vi "Sequencer.mqtt.vi"() -> ()   [LabVIEW 2014]
uses:
  <vilib>/daq.io/MQTT LabVIEW Client/Controls/Connection_Return_Codes.ctl
  <vilib>/addons/zeromq/socket_type.ctl
  <vilib>/daq.io/MQTT LabVIEW Client/Controls/Connect_Flags.ctl
  <vilib>/daq.io/MQTT LabVIEW Client/Controls/QoS.ctl
  <vilib>/daq.io/MQTT LabVIEW Client/Controls/DUP_Flag.ctl
  <vilib>/daq.io/MQTT LabVIEW Client/Controls/Retain_Flag.ctl
  <vilib>/Analysis/NI_AALPro.lvlib
  <vilib>/addons/zeromq/zmq_context.lvclass
  <vilib>/addons/zeromq/zmq_socket.lvclass
  <vilib>/addons/zeromq/zeromq.lvlib
  <vilib>/daq.io/MQTT LabVIEW Client/MQTT_Functions.lvlib
panel:
  out "MQTT Error":string
  out "MQTT Status":T1=enum."Connection refused: not authorized"
  out "Counts":u32[](array[numeric])
  out "PMT4":u32[](array[numeric])
  out "PMT3":u32[](array[numeric])
  out "PMT2":u32[](array[numeric])
  out "PMT1":u32[](array[numeric])
  in  "Threshold":dbl=1.0
  out "CompiledSequence":string="#DopplerCooling\r\n0.9 10100000 00000000 00000000\r\n\r\n#Pump\r\n0.3 01000000 00000000 00000000\r\n\r\n#Pulsed\r\n0.2 00100000 00000000 00000000\r\n0.4 00000100 00000000 00000000\r\n0.2 00000000 10000000 00000000\r\n0.2 01000000 00000000 01000000\n"
  out "ChapterNames":string[](array[string])
  out "ChapterPositions":u32[](array[numeric])
  in  "Scan":enum32{"Time"}(tab)
  out "Now (us)":dbl=1.0 format="%.2f"
  in  "Step (us)":dbl=1.0 format="%.2f"
  in  "End (us)":dbl=1.0 format="%.2f"
  in  "Start (us)":dbl=1.0 format="%.2f"
  in  "Time Scan":bool
  in  "Chapter":u16(ring) items=["Zero", "DopplerCooling[0]", "DopplerCooling[1]", "DopplerCooling[2]", "Zero"]
  in  "Once":bool=TRUE
  in  "Sequencer Port":refnum<visa-resource-name>="COM8"
  in  "Send":bool
  out "Durations Backup":dbl[](array[numeric])
  out "Durations":dbl[](array[numeric])
  in  "Period (ns)":dbl=5.0
  out "States":string[](array[string])
  in  "Sequencer":bool
  in  "Edit":enum32{"Sequence"}(tab)
  in  "Sequence":string
  in  "Save":bool
  in  "Chapter (us)":string
  in  "Sequence File":path=path "D:/Data/Sequence/Cooling.seq"
  in  "Repeats":u32=100
  in  "Compile":bool
  in  "Data":bool
  out "Clock":string
  in  "Detect":enum32{"PMT", "TTL"}(tab)
  in  "4":bool
  in  "3":bool
  in  "2":bool
  in  "1":bool=TRUE
  in  "Save":bool
  in  "Count or State":i16(ring) items=["Count", "State"]
  in  "Fit":bool
  out "Peak":u32
  out "?":cluster{dbl[], "Axis":dbl[]}(graph)
  out "?":cluster{"Axis":dbl[], "Histogram":i32[]}(graph)
  in  "Data Chapter":i16(ring) items=["All", "DopplerCooling[2]"]
  out "Average Counts or States":dbl(graph)
  out "Average of Scans":dbl[](graph)
  out "data file":string
  out "History Data":dbl[](array[numeric])
  in  "Sweep":bool
  out "Digital Waveform Graph":digitaldata(graph)
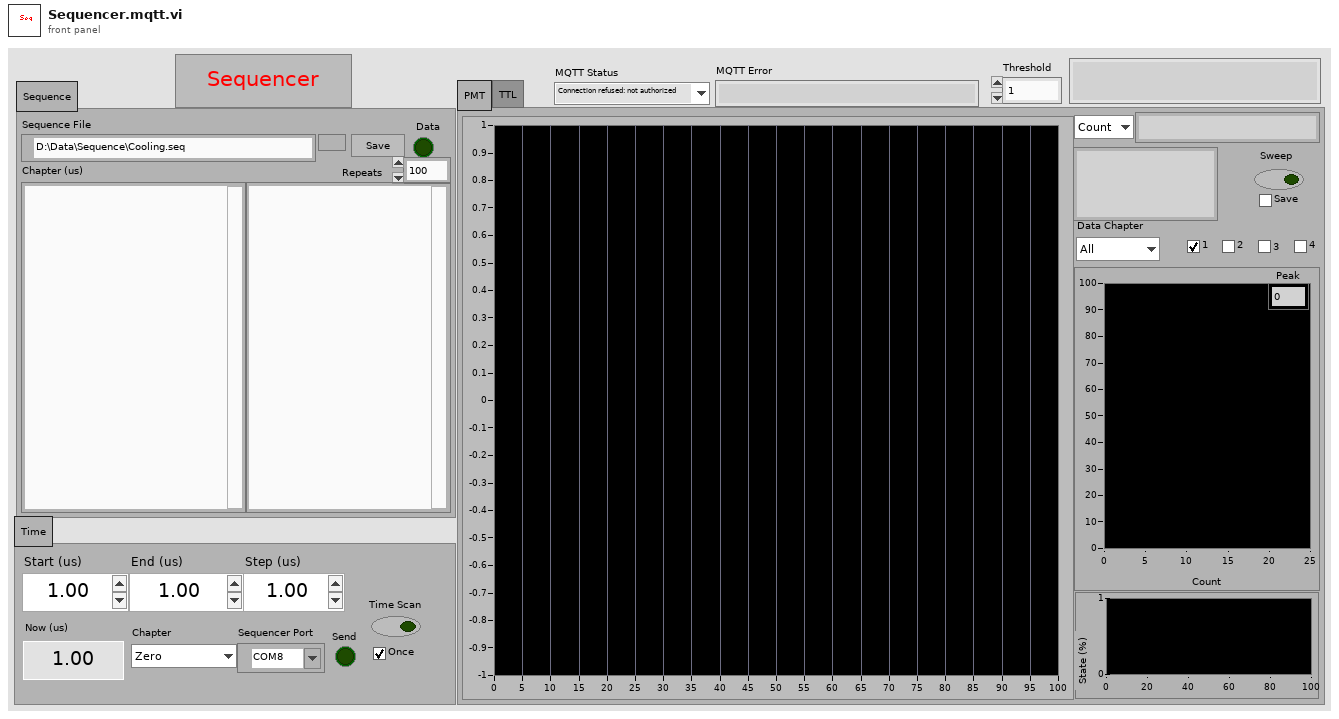
[diagram p1: front panel]
types:
  T1 = typedef "MQTT_Functions.lvlib/Connection_Return_Codes.ctl" = enum16{"Connection accepted", "Connection refused: unacceptable protocol version", "Connection refused: identifier rejected", "Connection refused: Server unavailable", "Connection refused: bad user name or password", "Connection refused: not authorized"}
  T2 = typedef "MQTT_Functions.lvlib/QoS.ctl" = enum8{"At most once", "At least once", "Exactly once", "Reserved"}
  T3 = typedef "MQTT_Functions.lvlib/DUP_Flag.ctl" = bool
  T4 = typedef "MQTT_Functions.lvlib/Retain_Flag.ctl" = bool
  T5 = cluster{"QoS":T2, "DUP":T3, "Retain":T4, "Keep Alive (sec)":u16}
  T6 = typedef "MQTT_Functions.lvlib/Connect_Flags.ctl" = cluster{"user name":bool, "password":bool, "will retain":bool, "will flag":bool, "clean session":bool, "reserved":bool, "will QoS":T2}
  T7 = typedef "zeromq.lvlib/socket_type.ctl" = enum8{"ZMQ_PAIR", "ZMQ_PUB", "ZMQ_SUB", "ZMQ_REQ", "ZMQ_REP", "ZMQ_DEALER", "ZMQ_ROUTER", "ZMQ_PULL", "ZMQ_PUSH", "ZMQ_XPUB", "ZMQ_XSUB"}
  T8 = cluster{"lower":dbl, "upper":dbl, "inclusion":enum32{"lower", "upper", "both", "neither"}}[]
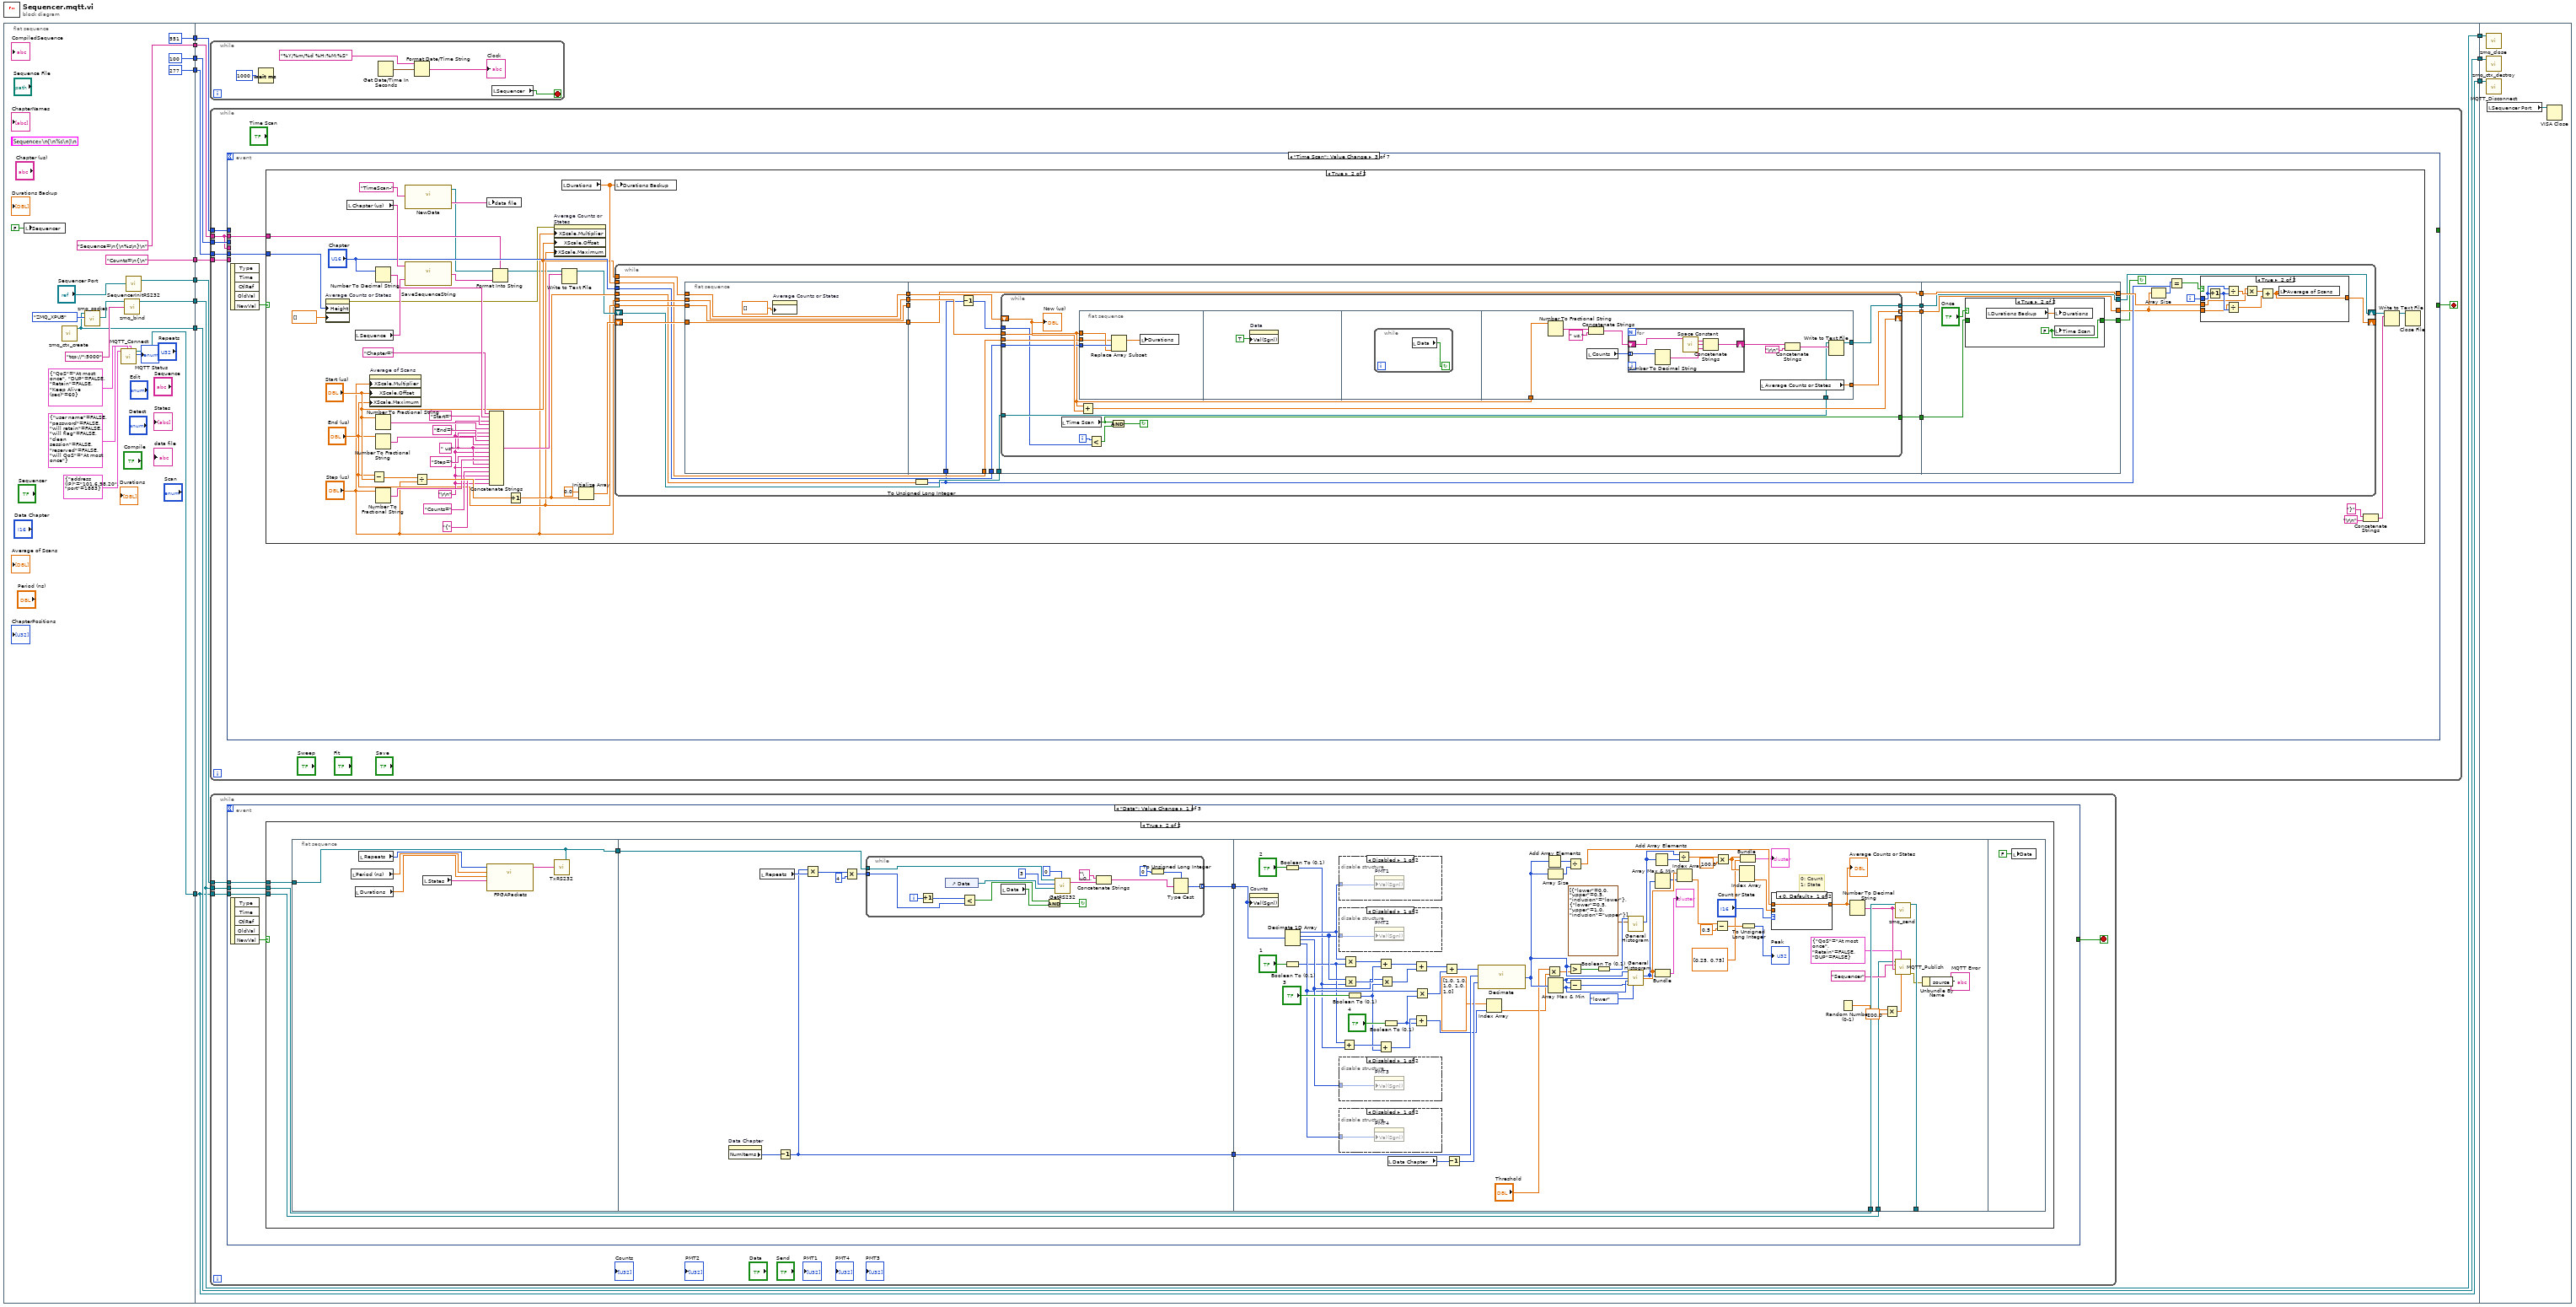
[diagram p0: block diagram]
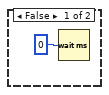
[diagram p2: hidden frame]
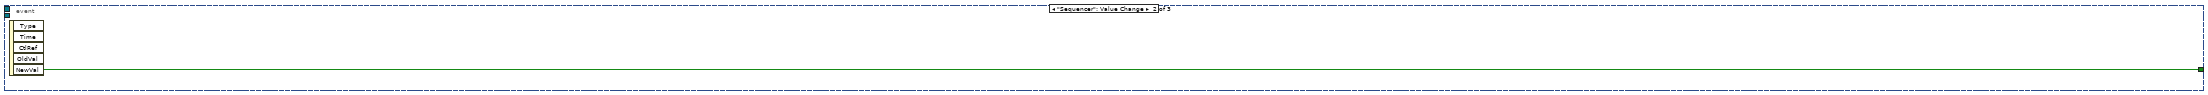
[diagram p8: hidden frame]
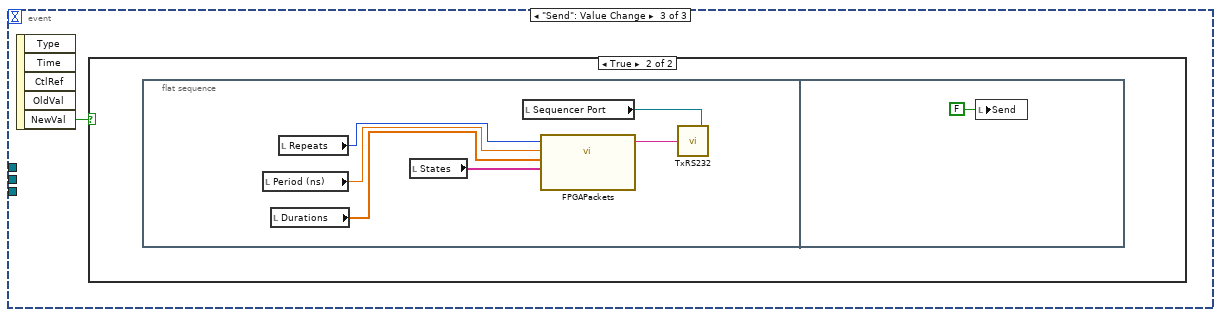
[diagram p9: hidden frame]
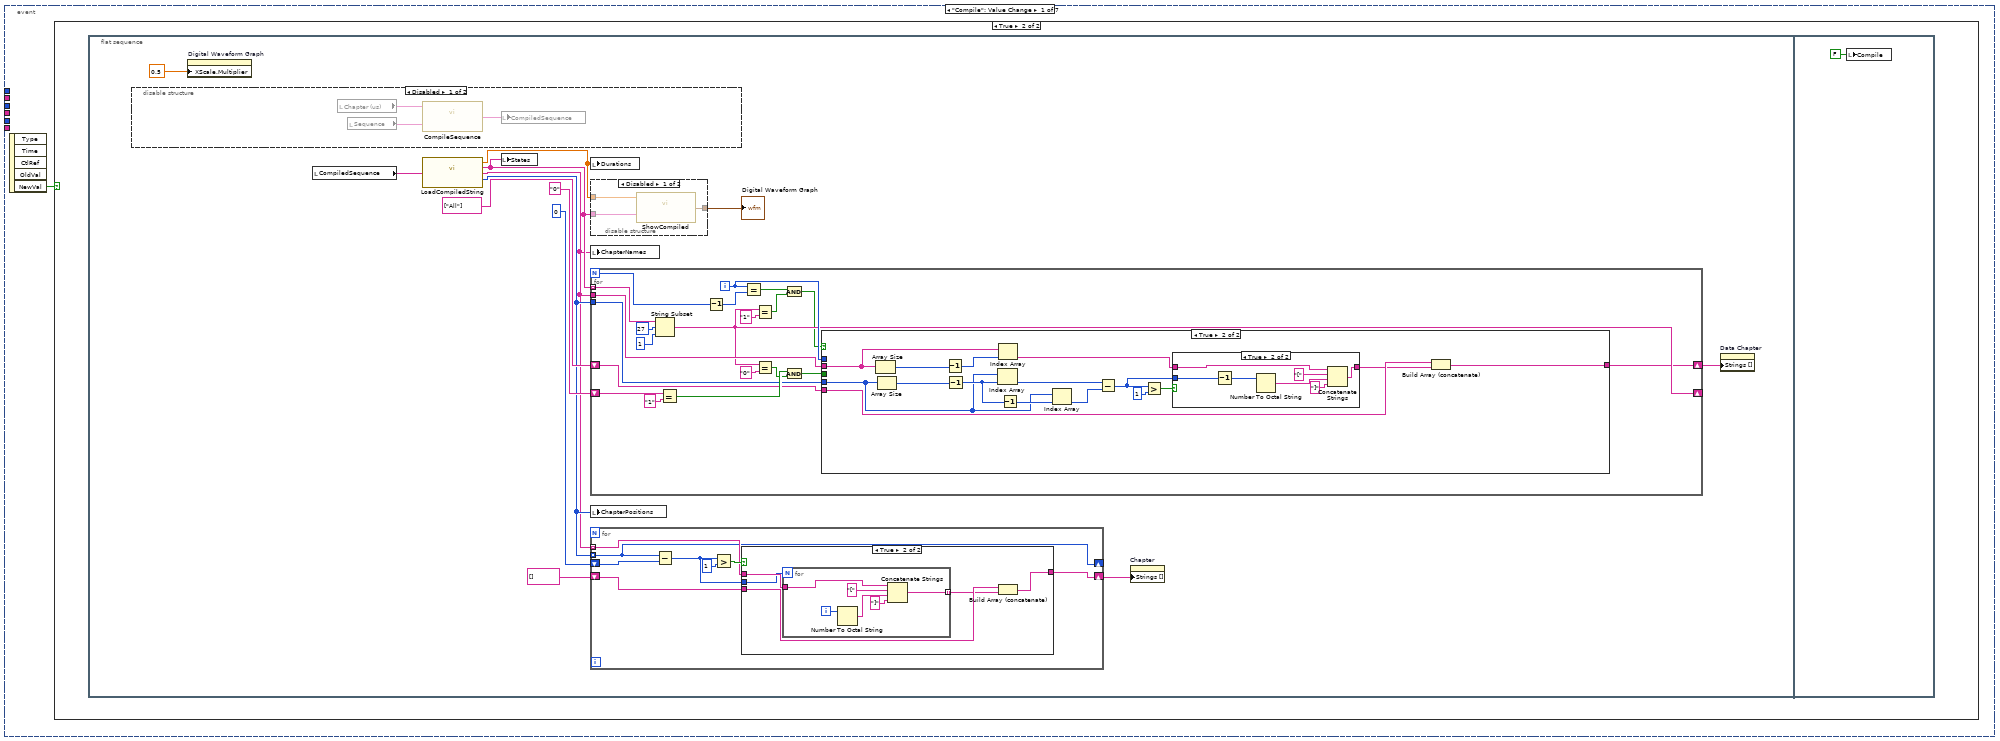
[diagram p11: hidden frame]
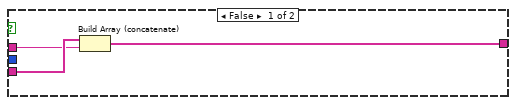
[diagram p15: hidden frame]
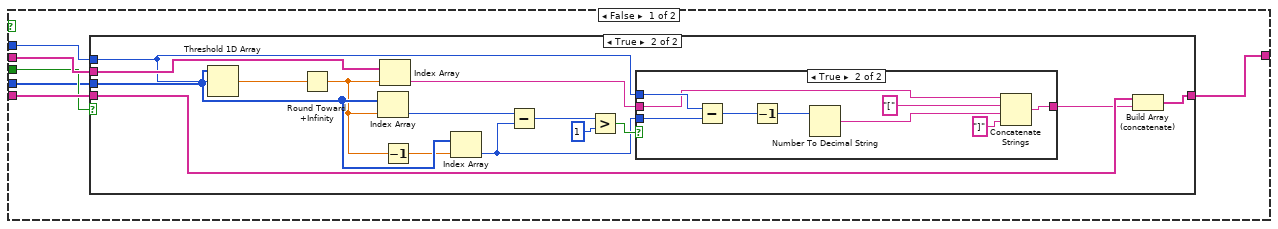
[diagram p16: hidden frame]
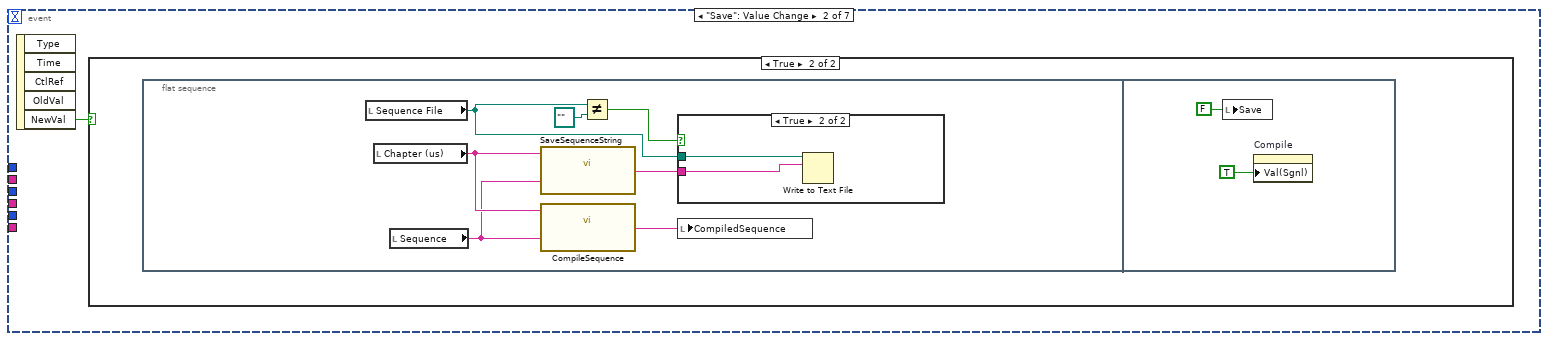
[diagram p20: hidden frame]
diagram:
  n1 = flat-sequence {
    tunnel: [w23] -> w12
    tunnel: [u32 277 ("XControl:Container Bounds:Height")] -> w11
    tunnel: [u32 551 ("Plot Area:Size:Height")] -> w10
    tunnel: [100 ("y")] -> w9
    tunnel: ["Sequence=\n{\n%s\n}\n" ("format string")] -> w8
    tunnel: ["Counts=\n{\n" ("text")] -> w7
    tunnel: [w19] -> w6
    tunnel: [w18] -> w3
    tunnel: [w16] -> w2
    tunnel: w12 -> [w39]
    tunnel: w11 -> [w38]
    tunnel: w10 -> [w37]
    tunnel: w9 -> [w36]
    tunnel: w8 -> [w35]
    tunnel: w7 -> [w34]
    tunnel: w6 -> [w32]
    tunnel: [w32] -> w5
    tunnel: [w33] -> w4
    tunnel: w3 -> [w33]
    tunnel: w2 -> [w31]
    tunnel: [w31] -> w1
    tunnel: w5 -> [w534]
    tunnel: w4 -> [w533]
    tunnel: w1 -> [w532]
    frame #0 {
      n2 = local write "Sequencer"(FALSE ("Sequencer")) -> ()
      n3 = call <vilib>:"zmq_ctx_create.vi"() -> ("context out"=w18:refnum<class "zmq_context.lvclass">)  [unwired: 4 in, 1 out]
      n4 = call <vilib>:"zmq_socket.vi"("socket type"=socket_type."ZMQ_XPUB", "context in"=w18) -> ("socket out"=w21:refnum<class "zmq_socket.lvclass">)  [unwired: 3 in, 2 out]
      n5 = call <vilib>:"MQTT_Connect.vi"("Connect Meta"=T5 {"QoS"=enum."At most once", "DUP"=FALSE, "Retain"=FALSE, "Keep Alive (sec)"=60}, "Connect Flags"=T6 {"user name"=FALSE, "password"=FALSE, "will retain"=FALSE, "will flag"=FALSE, "clean session"=FALSE, "reserved"=FALSE, "will QoS"=enum."At most once"}, "MQTT Broker"=cluster{"address (IP)":string, "port":u16} {"address (IP)"="101.6.98.20", "port"=1883}) -> ("Connection Status"=→"MQTT Status":T1, "connection ID out"=w16:refnum<k5>)  [unwired: 6 in, 1 out]
      n6 = call <vilib>:"zmq_bind.vi"("endpoint"="tcp://*:5000", "socket in"=w21) -> ("socket out"=w19:refnum<class "zmq_socket.lvclass">)  [unwired: 2 in, 1 out]
      n7 = call "SequencerInitRS232.vi"("VISA resource name"="Sequencer Port") -> ("reference out"=w23:refnum<visa-resource-name>)  [unwired: 1 out]
    }
    frame #1 {
      n8 = while {
        stop <- w40 stop-if-true
        n9 = Wait (ms)(milliseconds to wait=u32 1000) -> ()  [unwired: 1 out]
        n10 = Get Date/Time In Seconds() -> (seconds since 1Jan1904=w44:timestamp)
        n11 = Format Date/Time String(time format string (%c)="%Y/%m/%d %H:%M:%S", seconds (now)=w44) -> (date/time string=→"Clock":string)  [unwired: 1 in]
        n12 = local read "Sequencer"() -> (w40:bool)
      }
      n13 = while {
        tunnel: w38 -> [w180]
        tunnel: w37 -> [w179]
        tunnel: w36 -> [w178]
        tunnel: w35 -> [w176]
        tunnel: w34 -> [w177]
        stop <- w181 stop-if-true
        n14 = event shown="[2] \"Time Scan\": Value Change" {
          selector: _ -> [_ _ _ _ _ _ _]
          dyn-events: _ -> [_ _ _ _ _ _ _]
          timeout: _ -> [_ _ _ _ _ _ _]
          tunnel: [_ _ _ _ _ _ w531] -> _
          tunnel: [_ _ _ _ _ _ w531] -> w181
          tunnel: w180 -> [_ _ w315 _ _ _ _]
          tunnel: w179 -> [_ _ _ _ _ w468 _]
          tunnel: w178 -> [_ _ _ _ _ w467 _]
          tunnel: w176 -> [_ _ _ _ _ w466 _]
          tunnel: w177 -> [_ _ _ _ _ w465 _]
          tunnel: w176 -> [_ _ w314 _ _ _ _]
          event "Compile": Value Change {
            n15 = event-data() -> ("NewVal"=w182:bool)  [unwired: 1 in, 4 out]
            n16 = case shown="True" w182 {
              frame False {
              }
              frame True {
                n17 = flat-sequence {
                  frame #0 {
                    n18 = disable-structure shown="Disabled" {
                      frame Disabled {
                        n19 = local read "Chapter (us)"() -> (w201:string)
                        n20 = local read "Sequence"() -> (w200:string)
                        n21 = call "CompileSequence.vi"("Sequence"=w200, "Chapter"=w201) -> ("Compiled Sequence"=w199:string)
                        n22 = local write "CompiledSequence"(w199) -> ()
                      }
                      frame Enabled {
                      }
                    }
                    n23 = property on="Digital Waveform Graph" class="DigitalGraph (strict)"("XScale.Multiplier"=0.5 ("X Scale.Offset and Multiplier:Multiplier")) -> ()  [unwired: 2 in, 2 out]
                    n24 = local read "CompiledSequence"() -> (w183:string)
                    n25 = call "LoadCompiledString.vi"("Compiled String"=w183) -> ("Durations"=w194:dbl[], "States"=w193:string[], "ChapterNames"=w184:string[], "ChapterPositions"=w185:u32[])
                    n26 = local write "States"(w193) -> ()
                    n27 = local write "Durations"(w194) -> ()
                    n28 = disable-structure shown="Disabled" {
                      disable-tunnel: [w198 _] -> w195
                      disable-tunnel: w194 -> [w197 _]
                      disable-tunnel: w193 -> [w196 _]
                      frame Disabled {
                        n29 = call "ShowCompiled.vi"("States"=w196, "Durations"=w197) -> ("Digital Waveform Graph"=w198:digitaldata)
                      }
                      frame Enabled {
                      }
                    }
                    "Digital Waveform Graph" <- w195
                    n30 = local write "ChapterNames"(w184) -> ()
                    n31 = for {
                      N -> [w235]
                      tunnel: w193 -> [w244] mode=indexing
                      shift-right: [w232] -> _
                      shift-left: "0" -> [w242]
                      tunnel: w184 -> [w238]
                      shift-right: [w227] -> w188
                      shift-left: string[] ["All"] -> [w226]
                      tunnel: w185 -> [w225]
                      i -> [w236]
                      n32 = String Subset(string=w244, offset (0)=27, length (rest)=1 ("length (rest)")) -> (substring=w232:string)
                      n33 = Equal?(x=w242, y="1") -> (x = y?=w240:bool)
                      n34 = Decrement(x=w235) -> (x-1=w234:i32)
                      n35 = Equal?(x=w236, y=w234) -> (x = y?=w231:bool)
                      n36 = Equal?(x=w232, y="1") -> (x = y?=w230:bool)
                      n37 = Equal?(x=w232, y="0") -> (x = y?=w237:bool)
                      n38 = And(x=w231, y=w230) -> (x .and. y?=w229:bool)
                      n39 = And(x=w240, y=w237) -> (x .and. y?=w228:bool)
                      n40 = case shown="True" w229 {
                        tunnel: w238 -> [w250 w290]
                        tunnel: w226 -> [w249 w292]
                        tunnel: w236 -> [w248 _]
                        tunnel: w228 -> [w247 _]
                        tunnel: [w246 w291] -> w227
                        tunnel: w225 -> [w245 w284]
                        frame False {
                          n41 = case shown="True" w247 {
                            tunnel: w248 -> [_ w262]
                            tunnel: w250 -> [_ w263]
                            tunnel: w249 -> [w251 w265]
                            tunnel: [w251 w266] -> w246
                            tunnel: w245 -> [_ w259]
                            frame False {
                            }
                            frame True {
                              n42 = Threshold 1D Array(2:w262, 3:w259) -> (0:w264:dbl)  [unwired: 1 in]
                              n43 = Round Toward +Infinity(x=w264) -> (ceil(x): smallest int >= x=w257:dbl)
                              n44 = Index Array(array=w259, index=w257) -> (element=w256:u32)
                              n45 = Index Array(array=w263, index=w257) -> (element=w260:string)
                              n46 = Decrement(x=w257) -> (x-1=w258:dbl)
                              n47 = Index Array(array=w259, index=w258) -> (element=w252:u32)
                              n48 = Subtract(x=w256, y=w252) -> (x-y=w255:u32)
                              n49 = Greater?(x=w255, y=u32 1) -> (0:w253:bool)
                              n50 = case shown="True" w253 {
                                tunnel: w262 -> [_ w276]
                                tunnel: [w267 w270] -> w261
                                tunnel: w260 -> [w267 w269]
                                tunnel: w252 -> [_ w268]
                                frame False {
                                }
                                frame True {
                                n51 = Subtract(x=w276, y=w268) -> (x-y=w275:u32)
                                n52 = Decrement(x=w275) -> (x-1=w274:u32)
                                n53 = Number To Decimal String(number=w274) -> (decimal integer string=w271:string)  [unwired: 1 in]
                                n54 = Concatenate Strings(w269, "[" ("element"), w271, "]" ("element")) -> (w270:string)
                                }
                              }
                              n55 = Build Array (concatenate)(w265, w261) -> (w266:string[])
                            }
                          }
                        }
                        frame True {
                          n56 = Array Size(array=w290) -> (size(s)=w289:i32)
                          n57 = Array Size(array=w284) -> (size(s)=w287:i32)
                          n58 = Decrement(x=w289) -> (x-1=w288:i32)
                          n59 = Decrement(x=w287) -> (x-1=w286:i32)
                          n60 = Index Array(array=w284, index=w286) -> (element=w283:u32)
                          n61 = Index Array(array=w290, index=w288) -> (element=w279:string)
                          n62 = Decrement(x=w286) -> (x-1=w285:i32)
                          n63 = Index Array(array=w284, index=w285) -> (element=w282:u32)
                          n64 = Subtract(x=w283, y=w282) -> (x-y=w277:u32)
                          n65 = Greater?(x=w277, y=u32 1) -> (0:w280:bool)
                          n66 = case shown="True" w280 {
                            tunnel: w279 -> [w293 w300]
                            tunnel: [w293 w294] -> w278
                            tunnel: w277 -> [_ w297]
                            frame False {
                            }
                            frame True {
                              n67 = Decrement(x=w297) -> (x-1=w296:u32)
                              n68 = Number To Octal String(2:w296) -> (0:w295:string)  [unwired: 1 in]
                              n69 = Concatenate Strings(w300, "[" ("string"), w295, "]" ("string")) -> (w294:string)
                            }
                          }
                          n70 = Build Array (concatenate)(w292, w278) -> (w291:string[])
                        }
                      }
                    }
                    n71 = local write "ChapterPositions"(w185) -> ()
                    n72 = for {
                      tunnel: w185 -> [w202] mode=indexing
                      tunnel: w184 -> [w203] mode=indexing
                      shift-right: [w202] -> _
                      shift-left: u32 0 ("initial scan location") -> [w209]
                      shift-right: [w204] -> w190
                      shift-left: string[] [] -> [w205]
                      n73 = Subtract(x=w202, y=w209) -> (x-y=w206:u32)
                      n74 = Greater?(x=w206, y=u32 1) -> (0:w208:bool)
                      n75 = case shown="True" w208 {
                        tunnel: w203 -> [w211 w217]
                        tunnel: w206 -> [_ w216]
                        tunnel: w205 -> [w212 w215]
                        tunnel: [w210 w213] -> w204
                        frame False {
                          n76 = Build Array (concatenate)(w212, w211) -> (w210:string[])
                        }
                        frame True {
                          n77 = for {
                            N: w216 -> [_]
                            tunnel: w217 -> [w222]
                            tunnel: [w221] -> w214 mode=indexing
                            i -> [w223]
                            n78 = Number To Octal String(2:w223) -> (0:w220:string)  [unwired: 1 in]
                            n79 = Concatenate Strings(w222, "[" ("string"), w220, "]" ("string")) -> (w221:string)
                          }
                          n80 = Build Array (concatenate)(w215, w214) -> (w213:string[])
                        }
                      }
                    }
                    n81 = property on="Chapter" class="Ring (strict)"("Strings []"=w190) -> ()  [unwired: 2 in, 2 out]
                    n82 = property on="Data Chapter" class="Ring (strict)"("Strings []"=w188) -> ()  [unwired: 2 in, 2 out]
                  }
                  frame #1 {
                    n83 = local write "Compile"(FALSE ("Compile")) -> ()
                  }
                }
              }
            }
          }
          event "Save": Value Change {
            n84 = event-data() -> ("NewVal"=w302:bool)  [unwired: 1 in, 4 out]
            n85 = case shown="True" w302 {
              frame False {
              }
              frame True {
                n86 = flat-sequence {
                  frame #0 {
                    n87 = local read "Sequence File"() -> (w307:path)
                    n88 = local read "Chapter (us)"() -> (w305:string)
                    n89 = local read "Sequence"() -> (w304:string)
                    n90 = call "SaveSequenceString.vi"("Sequence"=w304, "Chapter"=w305) -> ("Sequence String"=w306:string)
                    n91 = call "CompileSequence.vi"("Sequence"=w304, "Chapter"=w305) -> ("Compiled Sequence"=w303:string)
                    n92 = Not Equal?(x=w307, y=path "") -> (x != y?=w309:bool)
                    n93 = case shown="True" w309 {
                      tunnel: w307 -> [_ w311]
                      tunnel: w306 -> [_ w310]
                      frame False {
                      }
                      frame True {
                        n94 = Write to Text File(file (use dialog)=w311, text=w310) -> ()  [unwired: 2 in, 3 out]
                      }
                    }
                    n95 = local write "CompiledSequence"(w303) -> ()
                  }
                  frame #1 {
                    n96 = local write "Save"(FALSE ("Compile")) -> ()
                    n97 = property on="Compile" class="Bool (strict)"("Val(Sgnl)"=TRUE ("Value (Signaling)")) -> ()  [unwired: 2 in, 2 out]
                  }
                }
              }
            }
          }
          event "Time Scan": Value Change {
            n98 = event-data() -> ("NewVal"=w316:bool)  [unwired: 1 in, 4 out]
            n99 = case shown="True" w316 {
              tunnel: w315 -> [_ w328]
              tunnel: w314 -> [_ w321]
              frame False {
                n100 = local read "Durations Backup"() -> (w317:dbl[])
                n101 = local write "Durations"(w317) -> ()
              }
              frame True {
                w341 = " us" ("string")
                w338 = "\r\n"
                n102 = property on="Average Counts or States" class="WFChart (strict)"("Height"=w328, "History Data"=dbl[] []) -> (error out=w327:errorcluster)  [unwired: 2 in, 1 out]
                n103 = local read "Chapter (us)"() -> (w348:string)
                n104 = local read "Sequence"() -> (w349:string)
                n105 = property on="Average of Scans" class="WFGraph (strict)"("XScale.Multiplier"="Step (us)", "XScale.Offset"="Start (us)", "XScale.Maximum"="End (us)") -> ()  [unwired: 2 in, 2 out]
                n106 = Subtract(x="End (us)", y="Start (us)") -> (x-y=w356:dbl)
                n107 = Number To Decimal String(number="Chapter") -> (decimal integer string=w352:string)  [unwired: 1 in]
                n108 = Number To Fractional String(number="Start (us)") -> (F-format string=w346:string)  [unwired: 3 in]
                n109 = Number To Fractional String(number="End (us)") -> (F-format string=w344:string)  [unwired: 3 in]
                n110 = Number To Fractional String(number="Step (us)") -> (F-format string=w342:string)  [unwired: 3 in]
                n111 = call "NewData.vi"("Prefix"="TimeScan-" ("string")) -> ("data file name"=w325:string, "data file refnum"=w319:refnum<file>)  [unwired: 2 in]
                n112 = call "SaveSequenceString.vi"("Sequence"=w349, "Chapter"=w348) -> ("Sequence String"=w320:string)
                n113 = Divide(x=w356, y="Step (us)") -> (x/y=w355:dbl)
                n114 = local write "data file"(w325) -> ()
                n115 = Concatenate Strings("Chapter=" ("string"), w352, w338, "Start=" ("string"), w346, w341, w338, "End=" ("string"), w344, w341, w338, "Step=" ("string"), w342, w341, w338, "Counts=" ("string"), w338, "{" ("string"), w338) -> (w350:string)
                n116 = Format Into String(format string=w321, initial string=w319, w320) -> (resulting string=w318:refnum<file>)  [unwired: 1 in, 1 out]
                n117 = Increment(x=w355) -> (x+1=w354:dbl)
                n118 = property on="Average Counts or States" class="WFChart (strict)"(error in=w327, "XScale.Multiplier"="Step (us)", "XScale.Offset"="Start (us)", "XScale.Maximum"="End (us)") -> ()  [unwired: 1 in, 2 out]
                n119 = local read "Durations"() -> (w331:dbl[])
                n120 = Write to Text File(file (use dialog)=w318, text=w350) -> (refnum out=w337:refnum<file>)  [unwired: 2 in, 2 out]
                n121 = Initialize Array(0.0 ("element"), w354) -> (w330:dbl[])
                n122 = local write "Durations Backup"(w331) -> ()
                n123 = while {
                  tunnel: "Start (us)" -> [w382]
                  tunnel: "Step (us)" -> [w381]
                  tunnel: "End (us)" -> [w380]
                  shift-right: [w370] -> _
                  shift-left: w330 -> [w379]
                  tunnel: w354 -> [w366]
                  tunnel: "Chapter" -> [w369]
                  shift-right: [w368] -> w335
                  shift-left: w337 -> [w367]
                  tunnel: w331 -> [w365]
                  i -> [w372]
                  stop <- w358 continue-if-true
                  n124 = flat-sequence {
                    tunnel: w379 -> [w393]
                    tunnel: w380 -> [w394]
                    tunnel: w381 -> [w395]
                    tunnel: w382 -> [w396]
                    tunnel: [w396] -> w378
                    tunnel: [w395] -> w377
                    tunnel: [w394] -> w376
                    tunnel: [w393] -> w375
                    tunnel: w378 -> [w407]
                    tunnel: w377 -> [w406]
                    tunnel: w376 -> [_]
                    tunnel: w375 -> [w405]
                    tunnel: w369 -> [w403]
                    tunnel: w367 -> [w402]
                    tunnel: w365 -> [w400]
                    tunnel: w364 -> [w399]
                    tunnel: [w405] -> w362
                    tunnel: [w404] -> w361
                    tunnel: [w401] -> w360
                    tunnel: [w397] -> w359
                    tunnel: [w446] -> w363
                    tunnel: [w447] -> w368
                    tunnel: [w443] -> w358
                    tunnel: [w448] -> w371
                    tunnel: w362 -> [w448]
                    tunnel: w361 -> [w444]
                    tunnel: w360 -> [w447]
                    tunnel: w359 -> [w446]
                    frame #0 {
                      n125 = property on="Average Counts or States" class="WFChart (strict)"("History Data"=dbl[] []) -> ()  [unwired: 2 in, 2 out]
                    }
                    frame #1 {
                      n126 = Decrement(x=w399) -> (x-1=w398:u32)
                      n127 = while {
                        shift-right: [w420] -> _
                        shift-left: w407 -> [w408]
                        tunnel: w406 -> [w418]
                        tunnel: [w417] -> w404
                        tunnel: w403 -> [w414]
                        tunnel: w402 -> [w415]
                        tunnel: [w416] -> w401
                        tunnel: w400 -> [w413]
                        tunnel: w398 -> [w410]
                        tunnel: [w409] -> w397 mode=indexing
                        i -> [w412]
                        stop <- w419 continue-if-true
                        n128 = local read "Time Scan"() -> (w417:bool)
                        n129 = flat-sequence {
                          tunnel: w414 -> [w424]
                          tunnel: w408 -> [w423]
                          tunnel: w413 -> [w421]
                          tunnel: w408 -> [w435]
                          tunnel: w415 -> [w430]
                          tunnel: [w429] -> w416
                          tunnel: [w427] -> w409
                          frame #0 {
                            n130 = Replace Array Subset(array=w421, new element=w423, index=w424) -> (w422:dbl[])
                            n131 = local write "Durations"(w422) -> ()
                          }
                          frame #1 {
                            n132 = property on="Data" class="Bool (strict)"("Val(Sgnl)"=TRUE ("Acquisition")) -> ()  [unwired: 2 in, 2 out]
                          }
                          frame #2 {
                            n133 = while {
                              stop <- w426 continue-if-true
                              n134 = local read "Data"() -> (w426:bool)
                            }
                          }
                          frame #3 {
                            n135 = Number To Fractional String(number=w435) -> (F-format string=w437:string)  [unwired: 3 in]
                            n136 = local read "Counts"() -> (w428:u32[])
                            n137 = Concatenate Strings(w437, " us," ("string")) -> (w434:string)
                            n138 = for {
                              tunnel: w428 -> [w442] mode=indexing
                              shift-right: [w440] -> w431
                              shift-left: w434 -> [w439]
                              n139 = Number To Decimal String(number=w442) -> (decimal integer string=w441:string)  [unwired: 1 in]
                              n140 = call <vilib>:"Space Constant.vi"() -> ("String"=w438:string)
                              n141 = Concatenate Strings(w439, w438, w441) -> (w440:string)
                            }
                            n142 = local read "Average Counts or States"() -> (w427:dbl)
                            n143 = Concatenate Strings(w431, "\r\n") -> (w432:string)
                            n144 = Write to Text File(file (use dialog)=w430, text=w432) -> (refnum out=w429:refnum<file>)  [unwired: 2 in, 2 out]
                          }
                        }
                        n145 = Add(x=w408, y=w418) -> (x+y=w420:dbl)
                        n146 = Less?(x=w412, y=w410) -> (x < y?=w411:bool)
                        n147 = And(x=w417, y=w411) -> (x .and. y?=w419:bool)
                        "Now (us)" <- w408
                      }
                    }
                    frame #2 {
                      n148 = case shown="True" "Once" {
                        tunnel: w444 -> [w449 _]
                        tunnel: [w449 w451] -> w443
                        frame False {
                        }
                        frame True {
                          w451 = FALSE ("Time Scan")
                          n149 = local read "Durations Backup"() -> (w450:dbl[])
                          n150 = local write "Durations"(w450) -> ()
                          n151 = local write "Time Scan"(w451) -> ()
                        }
                      }
                    }
                  }
                  n152 = To Unsigned Long Integer(number=w366) -> (unsigned 32bit integer=w364:u32)
                  n153 = Array Size(array=w363) -> (size(s)=w373:i32)
                  n154 = Equal?(x=w373, y=w364) -> (x = y?=w374:bool)
                  n155 = case shown="True" w374 {
                    tunnel: w372 -> [_ w387]
                    tunnel: w363 -> [_ w386]
                    tunnel: w371 -> [w383 w385]
                    tunnel: [w383 w384] -> w370
                    frame False {
                    }
                    frame True {
                      n156 = Increment(x=w387) -> (x+1=w390:i32)
                      n157 = Divide(x=w387, y=w390) -> (x/y=w388:dbl)
                      n158 = Divide(x=w386, y=w390) -> (x/y=w391:dbl[])
                      n159 = Multiply(x=w385, y=w388) -> (x*y=w389:dbl[])
                      n160 = Add(x=w389, y=w391) -> (x+y=w384:dbl[])
                      n161 = local write "Average of Scans"(w384) -> ()
                    }
                  }
                }
                n162 = Concatenate Strings("}" ("string"), "\r\n") -> (w332:string)
                n163 = Write to Text File(file (use dialog)=w335, text=w332) -> (refnum out=w336:refnum<file>)  [unwired: 2 in, 2 out]
                n164 = Close File(refnum=w336) -> ()  [unwired: 1 in, 2 out]
              }
            }
          }
          event "Fit": Value Change {
            n165 = event-data() -> ("NewVal"=w452:bool)  [unwired: 1 in, 4 out]
            n166 = case shown="True" w452 {
              frame False {
              }
              frame True {
                n167 = local write "Fit"(FALSE ("Fit")) -> ()
                n168 = property on="Average Counts or States" class="WFChart (strict)"() -> ("History Data"=→"History Data":dbl[])  [unwired: 2 in, 2 out]
              }
            }
          }
          event "Sequence File": Value Change {
            n169 = event-data() -> ("NewVal"=w456:path)  [unwired: 1 in, 4 out]
            n170 = call <vilib>:"Check if File or Folder Exists.vi"("path"=w456) -> ("file or folder exists?"=w457:bool, "dup path"=w455:path)  [unwired: 8 in, 1 out]
            n171 = case shown="True" w457 {
              tunnel: w455 -> [_ w458]
              frame False {
              }
              frame True {
                n172 = flat-sequence {
                  tunnel: w458 -> [w462]
                  frame #0 {
                    n173 = Read from Text File(file (use dialog)=w462) -> (text=w463:string)  [unwired: 3 in, 3 out]
                    n174 = call "LoadSequenceString.vi"("Sequence String"=w463) -> ("Chapter"=w461:string, "Sequence"=w460:string)
                    n175 = local write "Chapter (us)"(w461) -> ()
                    n176 = call "CompileSequence.vi"("Sequence"=w460, "Chapter"=w461) -> ("Compiled Sequence"=w459:string)
                    n177 = local write "Sequence"(w460) -> ()
                    n178 = local write "CompiledSequence"(w459) -> ()
                  }
                  frame #1 {
                    n179 = property on="Compile" class="Bool (strict)"("Val(Sgnl)"=TRUE ("Value (Signaling)")) -> ()  [unwired: 2 in, 2 out]
                  }
                }
              }
            }
          }
          event "Sweep": Value Change {
            n180 = event-data() -> ("NewVal"=w469:bool)  [unwired: 1 in, 4 out]
            n181 = case shown="True" w469 {
              tunnel: w468 -> [_ w474]
              tunnel: w467 -> [_ _]
              tunnel: w466 -> [_ w473]
              tunnel: w465 -> [_ w472]
              frame False {
              }
              frame True {
                n182 = flat-sequence {
                  tunnel: w474 -> [w484]
                  tunnel: w473 -> [w479]
                  tunnel: w472 -> [w478]
                  tunnel: [w477] -> w471
                  tunnel: ["Save"] -> w470
                  tunnel: w471 -> [w501]
                  tunnel: w470 -> [w499]
                  frame #0 {
                    w485 = dbl[] [] ("History Data")
                    w482 = 0.0 ("X Scale.Offset and Multiplier:Offset")
                    w483 = 1.0 ("X Scale.Offset and Multiplier:Multiplier")
                    n183 = property on="Average Counts or States" class="WFChart (strict)"("History Data"=w485, "Height"=w484) -> (error out=w480:errorcluster)  [unwired: 2 in, 1 out]
                    n184 = property on="Average of Scans" class="WFGraph (strict)"("XScale.Multiplier"=w483, "XScale.Offset"=w482, "XScale.Maximum"=0.0 ("X Scale.Range:Maximum"), "Value"=w485) -> ()  [unwired: 2 in, 2 out]
                    n185 = case shown="True" "Save" {
                      tunnel: ["" w496] -> w476
                      tunnel: w479 -> [_ w493]
                      tunnel: w478 -> [_ w490]
                      tunnel: [_ w489] -> w477
                      frame False {
                      }
                      frame True {
                        n186 = local read "Chapter (us)"() -> (w495:string)
                        n187 = local read "Sequence"() -> (w491:string)
                        n188 = call "NewData.vi"("Prefix"="Sweep-") -> ("data file name"=w496:string, "data file refnum"=w494:refnum<file>)  [unwired: 2 in]
                        n189 = call "SaveSequenceString.vi"("Sequence"=w491, "Chapter"=w495) -> ("Sequence String"=w492:string)
                        n190 = Format Into String(format string=w493, initial string=w494, w492) -> (resulting string=w488:refnum<file>)  [unwired: 1 in, 1 out]
                        n191 = Write to Text File(file (use dialog)=w488, text=w490) -> (refnum out=w489:refnum<file>)  [unwired: 2 in, 2 out]
                      }
                    }
                    n192 = property on="Average Counts or States" class="WFChart (strict)"(error in=w480, "XScale.Multiplier"=w483, "XScale.Offset"=w482, "XScale.Maximum"=100.0 ("X Scale.Range:Maximum")) -> ()  [unwired: 1 in, 2 out]
                    n193 = local write "data file"(w476) -> ()
                  }
                  frame #1 {
                    n194 = while {
                      tunnel: [w508] -> w500
                      tunnel: w501 -> [w507]
                      tunnel: w499 -> [w506]
                      tunnel: [w506] -> w498
                      i -> [w505]
                      stop <- w509 continue-if-true
                      n195 = flat-sequence {
                        tunnel: [w515] -> w508
                        tunnel: w507 -> [w514]
                        tunnel: w506 -> [w513]
                        tunnel: w505 -> [w512]
                        frame #0 {
                          n196 = property on="Data" class="Bool (strict)"("Val(Sgnl)"=TRUE ("Value (Signaling)")) -> ()  [unwired: 2 in, 2 out]
                        }
                        frame #1 {
                          n197 = while {
                            stop <- w511 continue-if-true
                            n198 = local read "Data"() -> (w511:bool)
                          }
                        }
                        frame #2 {
                          n199 = case shown="True" w513 {
                            tunnel: [w516 w521] -> w515
                            tunnel: w514 -> [w516 w520]
                            tunnel: w512 -> [_ w517]
                            frame False {
                            }
                            frame True {
                              n200 = local read "Counts"() -> (w525:u32[])
                              n201 = Format Into String(format string="%d One,", w517) -> (resulting string=w518:string)  [unwired: 2 in, 1 out]
                              n202 = for {
                                tunnel: w525 -> [w530] mode=indexing
                                shift-right: [w528] -> w524
                                shift-left: w518 -> [w527]
                                n203 = Number To Decimal String(number=w530) -> (decimal integer string=w529:string)  [unwired: 1 in]
                                n204 = call <vilib>:"Space Constant.vi"() -> ("String"=w526:string)
                                n205 = Concatenate Strings(w527, w526, w529) -> (w528:string)
                              }
                              n206 = Concatenate Strings(w524, "\r\n") -> (w522:string)
                              n207 = Write to Text File(file (use dialog)=w520, text=w522) -> (refnum out=w521:refnum<file>)  [unwired: 2 in, 2 out]
                            }
                          }
                        }
                      }
                      n208 = local read "Sweep"() -> (w509:bool)
                    }
                    n209 = case shown="True" w498 {
                      tunnel: w500 -> [_ w503]
                      frame False {
                      }
                      frame True {
                        n210 = Write to Text File(file (use dialog)=w503, text="}\n") -> (refnum out=w504:refnum<file>)  [unwired: 2 in, 2 out]
                        n211 = Close File(refnum=w504) -> ()  [unwired: 1 in, 2 out]
                      }
                    }
                  }
                }
              }
            }
          }
          event "Sequencer": Value Change {
            n212 = event-data() -> ("NewVal"=w531:bool)  [unwired: 1 in, 4 out]
          }
        }
      }
      n213 = while {
        tunnel: w39 -> [w48]
        tunnel: w32 -> [w46]
        tunnel: w31 -> [w45]
        stop <- w47 stop-if-true
        n214 = event shown="[0] \"Data\": Value Change" {
          selector: _ -> [_ _ _]
          dyn-events: _ -> [_ _ _]
          timeout: _ -> [_ _ _]
          tunnel: w48 -> [w52 _ _]
          tunnel: [_ w167 _] -> w47
          tunnel: w46 -> [w50 _ _]
          tunnel: w45 -> [w49 _ _]
          event "Data": Value Change {
            n215 = event-data() -> ("NewVal"=w51:bool)  [unwired: 1 in, 4 out]
            n216 = case shown="True" w51 {
              tunnel: w52 -> [_ w59]
              tunnel: w50 -> [_ w55]
              tunnel: w49 -> [_ w54]
              frame False {
                n217 = Wait (ms)(milliseconds to wait=u32 0) -> ()  [unwired: 1 out]
              }
              frame True {
                n218 = flat-sequence {
                  tunnel: w59 -> [w64]
                  tunnel: [w64] -> w56
                  tunnel: [w71] -> w58
                  tunnel: [w69] -> w57
                  tunnel: w56 -> [w73]
                  tunnel: w58 -> [w128]
                  tunnel: w57 -> [w134]
                  tunnel: w55 -> [w101]
                  tunnel: [w99] -> _
                  tunnel: w54 -> [w96]
                  frame #0 {
                    n219 = local read "Period (ns)"() -> (w62:dbl)
                    n220 = local read "Durations"() -> (w61:dbl[])
                    n221 = local read "Repeats"() -> (w63:u32)
                    n222 = local read "States"() -> (w60:string[])
                    n223 = call "FPGAPackets.vi"("Repeats"=w63, "Period (ns)"=w62, "Durations"=w61, "States"=w60) -> ("Packets"=w65:string)  [unwired: 1 in, 1 out]
                    n224 = call "TxRS232.vi"("VISA resource name"=w64, "Data"=w65) -> ()
                  }
                  frame #1 {
                    n225 = property on="Data Chapter" class="Ring (strict)"() -> ("NumItems"=w72:u32)  [unwired: 2 in, 2 out]
                    n226 = local read "Repeats"() -> (w70:u32)
                    n227 = Decrement(x=w72) -> (x-1=w69:u32)
                    n228 = Multiply(x=w69, y=w70) -> (x*y=w68:u32)
                    n229 = Multiply(x=w68, y=u32 4) -> (x*y=w67:u32)
                    n230 = while {
                      tunnel: w73 -> [w81]
                      tunnel: [w82] -> w71 mode=indexing
                      tunnel: w67 -> [w77]
                      i -> [w76]
                      stop <- w85 continue-if-true
                      n231 = Increment(x=w76) -> (x+1=w75:i32)
                      n232 = control-ref of="Data"() -> (w78:refnum<vi>)
                      n233 = Less?(x=w75, y=w77) -> (x < y?=w84:bool)
                      n234 = local read "Data"() -> (w86:bool)
                      n235 = And(x=w84, y=w86) -> (x .and. y?=w85:bool)
                      n236 = call "GetRS232.vi"("VISA resource name"=w81, "Bytes To Read"=3, "Control"=w78, "Limit"=0) -> ("Data"=w79:string)  [unwired: 1 in, 1 out]
                      n237 = Concatenate Strings("\u0000" ("string"), w79) -> (w83:string)
                      n238 = To Unsigned Long Integer(number=u32 0) -> (unsigned 32bit integer=w89:u32)
                      n239 = Type Cast(type=w89, x=w83) -> (*(type *) &x=w82:u32)
                    }
                  }
                  frame #2 {
                    # "0: Count\n1: State"
                    n240 = property on="Counts" class="Arr (strict)"("Val(Sgnl)"=w128) -> ()  [unwired: 2 in, 2 out]
                    n241 = Boolean To (0,1)(Boolean="2") -> (0, 1=w111:i16)
                    n242 = Boolean To (0,1)(Boolean="1") -> (0, 1=w112:i16)
                    n243 = Decimate 1D Array(w128) -> (w127:u32[], w124:u32[], w120:u32[], w117:u32[])
                    n244 = disable-structure shown="Disabled" {
                      disable-tunnel: w127 -> [w163 _]
                      frame Disabled {
                        n245 = property on="PMT1" class="Arr (strict)"("Val(Sgnl)"=w163) -> ()  [unwired: 2 in, 2 out]
                      }
                      frame Enabled {
                      }
                    }
                    n246 = disable-structure shown="Disabled" {
                      disable-tunnel: w124 -> [w162 _]
                      frame Disabled {
                        n247 = property on="PMT2" class="Arr (strict)"("Val(Sgnl)"=w162) -> ()  [unwired: 2 in, 2 out]
                      }
                      frame Enabled {
                      }
                    }
                    n248 = disable-structure shown="Disabled" {
                      disable-tunnel: w120 -> [w161 _]
                      frame Disabled {
                        n249 = property on="PMT3" class="Arr (strict)"("Val(Sgnl)"=w161) -> ()  [unwired: 2 in, 2 out]
                      }
                      frame Enabled {
                      }
                    }
                    n250 = disable-structure shown="Disabled" {
                      disable-tunnel: w117 -> [w160 _]
                      frame Disabled {
                        n251 = property on="PMT4" class="Arr (strict)"("Val(Sgnl)"=w160) -> ()  [unwired: 2 in, 2 out]
                      }
                      frame Enabled {
                      }
                    }
                    n252 = Add(x=w112, y=w111) -> (x+y=w110:i16)
                    n253 = Multiply(x=w127, y=w112) -> (x*y=w113:u32[])
                    n254 = Multiply(x=w124, y=w111) -> (x*y=w123:u32[])
                    n255 = Boolean To (0,1)(Boolean="3") -> (0, 1=w109:i16)
                    n256 = Add(x=w113, y=w123) -> (x+y=w118:u32[])
                    n257 = Add(x=w110, y=w109) -> (x+y=w108:i16)
                    n258 = Multiply(x=w120, y=w109) -> (x*y=w119:u32[])
                    n259 = Boolean To (0,1)(Boolean="4") -> (0, 1=w107:i16)
                    n260 = local read "Data Chapter"() -> (w132:i16)
                    n261 = Add(x=w118, y=w119) -> (x+y=w115:u32[])
                    n262 = Add(x=w108, y=w107) -> (x+y=w102:i16)
                    n263 = Multiply(x=w117, y=w107) -> (x*y=w116:u32[])
                    n264 = Add(x=w115, y=w116) -> (x+y=w114:u32[])
                    n265 = Decrement(x=w132) -> (x-1=w131:i16)
                    n266 = call "Decimate.vi"("i"=w131, "n"=w134, "Input Array"=w114) -> ("Decimated Array"=w156:u32[])
                    n267 = Index Array(array=dbl[] [1.0, 1.0, 1.0, 1.0, 1.0], index=w102) -> (element=w104:dbl)
                    n268 = Add Array Elements(numeric array=w156) -> (sum=w155:u32)
                    n269 = Multiply(x="Threshold", y=w104) -> (x*y=w103:dbl)
                    n270 = Array Size(array=w156) -> (size(s)=w154:i32)
                    n271 = Array Max & Min(array=w156) -> (max value=w135:u32, min value=w145:u32)  [unwired: 2 out]
                    n272 = Divide(x=w155, y=w154) -> (x/y=w158:dbl)
                    n273 = Greater?(x=w156, y=w103) -> (0:w141:bool[])
                    n274 = Subtract(x=w135, y=w145) -> (x-y=w144:u32)
                    n275 = Boolean To (0,1)(Boolean=w141) -> (0, 1=w140:i16[])
                    n276 = call <vilib>:"General Histogram.vi"("X"=w140, "Bins"=T8 [{"lower"=0.0, "upper"=0.5, "inclusion"=enum."lower"}, {"lower"=0.5, "upper"=1.0, "inclusion"=enum."upper"}]) -> ("Histogram"=w138:i32[])  [unwired: 9 in, 4 out]
                    n277 = call <vilib>:"General Histogram.vi"("X"=w156, "max"=w135, "min"=w145, "# bins"=w144, "inclusion"=enum32{"lower", "upper"}."lower") -> ("Histogram"=w146:i32[], "Axis"=w148:dbl[])  [unwired: 6 in, 3 out]
                    n278 = Add Array Elements(numeric array=w138) -> (sum=w139:i32)
                    n279 = Array Max & Min(array=w146) -> (max index (indices)=w147:i32)  [unwired: 3 out]
                    n280 = Bundle("Axis"=w148, "Histogram"=w146) -> (→"?":cluster{"Axis":dbl[], "Histogram":i32[]})  [unwired: 1 in]
                    n281 = Divide(x=w138, y=w139) -> (x/y=w136:dbl[])
                    n282 = Index Array(array=w148, index=w147) -> (element=w152:dbl)
                    n283 = Subtract(x=w152, y=0.5) -> (x-y=w151:dbl)
                    n284 = Multiply(x=w136, y=100.0) -> (x*y=w157:dbl[])
                    n285 = Index Array(array=w157) -> (element #2=w159:dbl)  [unwired: 2 in, 1 out]
                    n286 = Bundle(w157, "Axis"=dbl[] [0.25, 0.75]) -> (→"?":cluster{dbl[], "Axis":dbl[]})  [unwired: 1 in]
                    n287 = To Unsigned Long Integer(number=w151) -> (unsigned 32bit integer=→"Peak":u32)
                    n288 = case shown="0, Default" "Count or State" {
                      tunnel: w158 -> [w164 _]
                      tunnel: [w164 w165] -> w100
                      tunnel: w159 -> [_ w165]
                      frame 0, Default {
                      }
                      frame 1 {
                      }
                    }
                    "Average Counts or States" <- w100
                    n289 = Random Number (0-1)() -> (number: 0 to 1=w94:dbl)
                    n290 = Number To Decimal String(number=w100) -> (decimal integer string=w98:string)  [unwired: 1 in]
                    n291 = Multiply(x=w94, y=100.0) -> (x*y=w92:dbl)
                    n292 = call <vilib>:"zmq_send.vi"("data"=w98, "socket in"=w101) -> ("socket out"=w99:refnum<class "zmq_socket.lvclass">)  [unwired: 5 in, 1 out]
                    n293 = call <vilib>:"MQTT_Publish.vi"("Message ID"=w92, "Publish Meta"=cluster{"QoS":T2, "Retain":T4, "DUP":T3} {"QoS"=enum."At most once", "Retain"=FALSE, "DUP"=FALSE}, "Message to be published"=w98, "Topic"="Sequencer", "connection ID"=w96) -> ("error out"=w91:errorcluster)  [unwired: 5 in, 1 out]
                    n294 = Unbundle By Name(w91) -> ("source"=→"MQTT Error":string)
                  }
                  frame #3 {
                    n295 = local write "Data"(FALSE ("Acquisition")) -> ()
                  }
                }
              }
            }
          }
          event "Sequencer": Value Change {
            n296 = event-data() -> ("NewVal"=w167:bool)  [unwired: 1 in, 4 out]
          }
          event "Send": Value Change {
            n297 = event-data() -> ("NewVal"=w168:bool)  [unwired: 1 in, 4 out]
            n298 = case shown="True" w168 {
              frame False {
              }
              frame True {
                n299 = flat-sequence {
                  frame #0 {
                    n300 = local read "Period (ns)"() -> (w172:dbl)
                    n301 = local read "Durations"() -> (w170:dbl[])
                    n302 = local read "Repeats"() -> (w171:u32)
                    n303 = local read "States"() -> (w173:string[])
                    n304 = local read "Sequencer Port"() -> (w174:refnum<visa-resource-name>)
                    n305 = call "FPGAPackets.vi"("Repeats"=w171, "Period (ns)"=w172, "Durations"=w170, "States"=w173) -> ("Packets"=w169:string)  [unwired: 1 in, 1 out]
                    n306 = call "TxRS232.vi"("VISA resource name"=w174, "Data"=w169) -> ()
                  }
                  frame #1 {
                    n307 = local write "Send"(FALSE ("Send")) -> ()
                  }
                }
              }
            }
          }
        }
      }
    }
    frame #2 {
      n308 = call <vilib>:"zmq_close.vi"("socket"=w534) -> ()  [unwired: 4 in, 1 out]
      n309 = call <vilib>:"zmq_ctx_destroy.vi"("context in"=w533) -> ()  [unwired: 4 in, 1 out]
      n310 = call <vilib>:"MQTT_Disconnect.vi"("connection ID"=w532) -> ()  [unwired: 10 in, 1 out]
      n311 = local read "Sequencer Port"() -> (w535:refnum<visa-resource-name>)
      n312 = VISA Close(VISA resource name=w535) -> ()  [unwired: 1 in, 1 out]
    }
  }
